vi "MoveY.vi"(8 "error in (no error)":errorcluster, 10 "Up?":bool, 11 "PongPanel in":refnum<class "PongPanel.lvclass">) -> (0 "error out":errorcluster, 3 "PongPanel out":refnum<class "PongPanel.lvclass">)   [LabVIEW 2019, in "RT_Game.lvlib" / "PongPanel.lvclass"]
uses:
  PongPanel.lvclass
  C:/Users/FreshBob/Dropbox/VIs/myRIO_GameConsole/RT/RT_Game/GameObject/GameObject.lvclass
  GameObject/GameObject.lvclass/GameObject.ctl
  PongPanel.lvclass/PongPanel.ctl
  GameObject/Read position.vi
  GameObject/Read size.vi
  GameObject/Write position.vi
  Globals.vi
  RT_Game.lvlib
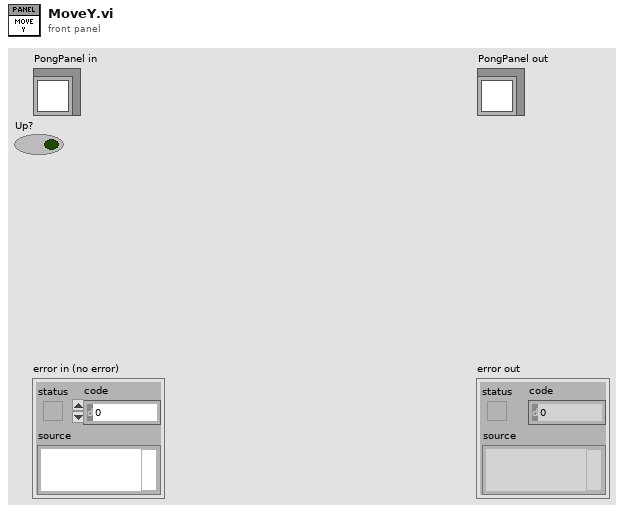
[diagram p1: front panel]
types:
  T1 = typedef "RT_Game.lvlib/Game.lvclass/Coordinate.ctl" = cluster{"x":dbl, "y":dbl}
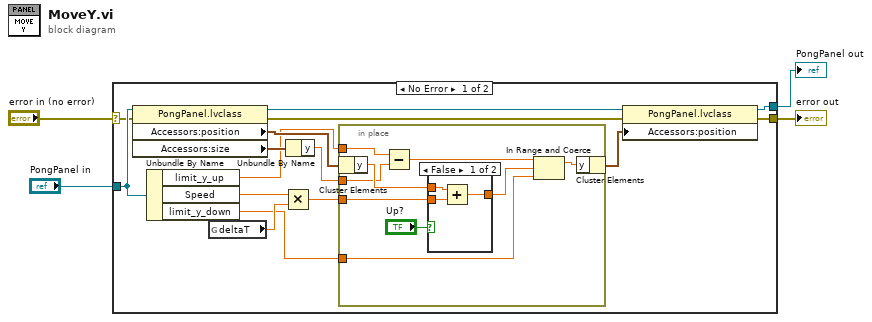
[diagram p0: block diagram]
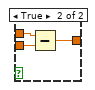
[diagram p2: hidden frame]
diagram:
  n1 = case shown="No Error" "error in (no error)" {
    selector: "error in (no error)" -> [w13 w36]
    tunnel: [w12 w36] -> w3
    tunnel: [w15 w35] -> w1
    tunnel: "PongPanel in" -> [w19 w35]
    frame No Error {
      n2 = property class="PongPanel.lvclass"(reference=w19, error in=w13) -> (reference out=w16:refnum<class "PongPanel.lvclass">, error out=w14:errorcluster, "Accessors:position"=w11:T1, "Accessors:size"=w8:T1)
      n3 = Unbundle By Name(w19) -> ("limit_y_up"=w7:dbl, "Speed"=w18:dbl, "limit_y_down"=w5:dbl)
      n4 = global read "Globals.vi" "deltaT"() -> (w17:dbl)
      n5 = Multiply(x=w18, y=w17) -> (x*y=w9:dbl)
      n6 = Unbundle By Name(w8) -> ("y"=w6:dbl)
      n7 = in-place {
        in-place-border: w9 -> [w27]
        in-place-border: w7 -> [w23]
        in-place-border: w6 -> [w22]
        in-place-border: w5 -> [w20]
        n8 = in-place-cluster #1(w11) -> ("y"=w28:dbl)
        n9 = Subtract(x=w23, y=w22) -> (x-y=w21:dbl)
        n10 = case shown="False" "Up?" {
          tunnel: w28 -> [w31 w34]
          tunnel: w27 -> [w30 w33]
          tunnel: [w29 w32] -> w26
          frame False {
            n11 = Add(x=w31, y=w30) -> (x+y=w29:dbl)
          }
          frame True {
            n12 = Subtract(x=w34, y=w33) -> (x-y=w32:dbl)
          }
        }
        n13 = In Range and Coerce(upper limit=w21, x=w26, lower limit=w20) -> (coerced(x)=w24:dbl)  [unwired: 1 out]
        n14 = in-place-cluster #1("y"=w24) -> (w10:T1)
      }
      n15 = property class="PongPanel.lvclass"(reference=w16, error in=w14, "Accessors:position"=w10) -> (reference out=w15:refnum<class "PongPanel.lvclass">, error out=w12:errorcluster)
    }
    frame Error {
    }
  }
  "error out" <- w3
  "PongPanel out" <- w1
